vi "get index by serial.vi"(8 "error in (no error)":errorcluster, 11 "Serial Number":string) -> (0 "error out":errorcluster, 3 "Index":i32)   [LabVIEW 2015, in "rtlsdr.lvlib"]
doc: "Get device index by USB serial string descriptor."
uses:
  rtlsdr.lvlib
  rtlsdr/rtlsdr.dll
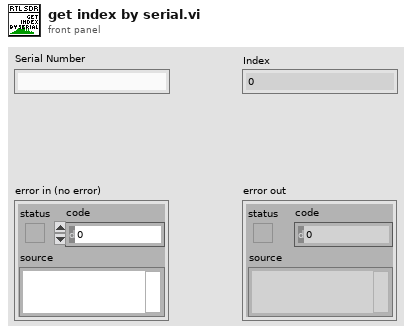
[diagram p1: front panel]
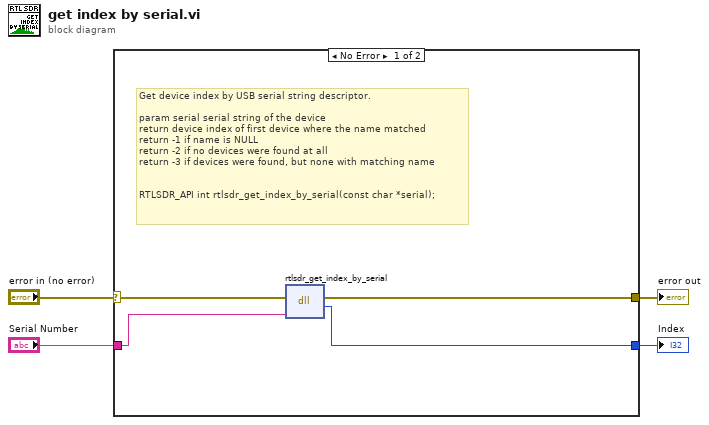
[diagram p0: block diagram]
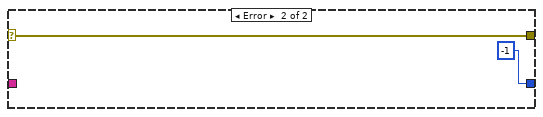
[diagram p2: hidden frame]
diagram:
  n1 = case shown="No Error" "error in (no error)" {
    selector: "error in (no error)" -> [w5 w10]
    tunnel: [w8 -1 ("return type")] -> w4
    tunnel: "Serial Number" -> [w7 _]
    tunnel: [w6 w10] -> w2
    frame No Error {
      # "Get device index by USB serial string descriptor.\n\nparam serial serial string of the device\nreturn device index of first device where the name matched\nreturn -1 if name is NULL\nreturn -2 if no devices were found at all\nreturn -3 if devices were found, but none with matching name\n\n\nRTLSDR_API int rtlsdr_get_index_by_serial(const char *serial);"
      n2 = dll-call lib="C:/Users/TheDoctor/Documents/Projects/Labview Libraries/rtlsdr/rtlsdr.*" fn="rtlsdr_get_index_by_serial"(error in=w5, "serial"=w7) -> (error out=w6:errorcluster, "return type"=w8:i32)  [unwired: 3 in, 1 out]
    }
    frame Error {
    }
  }
  "Index" <- w4
  "error out" <- w2
